vi "Add Data Sharing Framework with UDP Component to System Definition.vi"() -> ()   [LabVIEW 2017]
uses:
  DSF Core.lvlibp/Typedefs/DSF Engine Framework Configuration.ctl
  DSF Core.lvlibp/Typedefs/DSF Engine Plugin Configuration.ctl
  DSF Core.lvlibp/Typedefs/Core Plugin Configuration.ctl
  DSF Core.lvlibp/Typedefs/DSF Timing Info.ctl
  DSF Core.lvlibp/Typedefs/DSF Settings Info.ctl
  DSF Core.lvlibp/Typedefs/DSF Engine Plugin Thread Configuration.ctl
  DSF Core.lvlibp/Typedefs/Core Thread Configuration.ctl
  DSF Core.lvlibp/Typedefs/DSF Engine Transfer Group Configuration.ctl
  DSF Core.lvlibp/Typedefs/Core Group Configuration.ctl
  DSF Core.lvlibp/Typedefs/DSF Direction.ctl
  DSF Core.lvlibp/Typedefs/DSF Timeout Behavior.ctl
  DSF Core.lvlibp/Typedefs/DSF Engine Transfer Configuration.ctl
  DSF Core.lvlibp/Typedefs/Core Transfer Configuration.ctl
  DSF Core.lvlibp/Typedefs/DSF Engine Channel Configuration.ctl
  DSF Core.lvlibp/Typedefs/Core Channel Configuration.ctl
  DSF Core.lvlibp/Typedefs/DSF Data Type.ctl
  NationalInstruments.VeriStand.SystemDefinitionAPI
  DSF Core.lvlibp
  DSF Core.lvlibp/Classes/Configuration/Core/Channel/Channel Configuration.lvclass
  DSF Core.lvlibp/Classes/Configuration/Core/Transfer/Transfer Configuration.lvclass
  DSF Core.lvlibp/Classes/Configuration/Core/Group/Group Configuration.lvclass
  DSF Core.lvlibp/Classes/Configuration/Core/Thread/Thread Configuration.lvclass
  DSF Core.lvlibp/Classes/Configuration/Core/Plugin/Plugin Configuration.lvclass
  Scripting API/Data Sharing Framework Custom Device Scripting.lvlib
panel:
  in  "Launch Data Viewer":bool=TRUE
  in  "Data Server Frequency":dbl(ring)=10.0 items=["0.5 Hz"=0.5, "1.0 Hz"=1.0, "2.0 Hz"=2.0, "2.5 Hz"=2.5, "4.0 Hz"=4.0, "5.0 Hz"=5.0, "8.0 Hz"=8.0, "10.0 Hz"=10.0, "12.5 Hz"=12.5, "20.0 Hz"=20.0, "25.0 Hz"=25.0, "40.0 Hz"=40.0, "50.0 Hz"=50.0, "100.0 Hz"=100.0]
  in  "Enable Data Server":bool=TRUE
  in  "Channels":T1(array[cluster])
  in  "Output System Definition File":path=path "System Definition Files/DSF_UDP.nivssdf"
  in  "Input System Definition File":path=path "System Definition Files/DSF_empty.nivssdf"
  # "Overview: Demonstrates using the Data Sharing Framework scripting API to add a UDP plugin for data communication. \n\nInstructions:\n1. Per your application requirements, configure the data block to share.\n2. Browse to a path to save the system definition file as the output Output System Definition File.  This may be the same as the input file.\n3. Run the VI and verify its results."
  # "Configure Data Server for Validation"
  # "Data Sharing Framework Channels"
  # "System Definition Files"
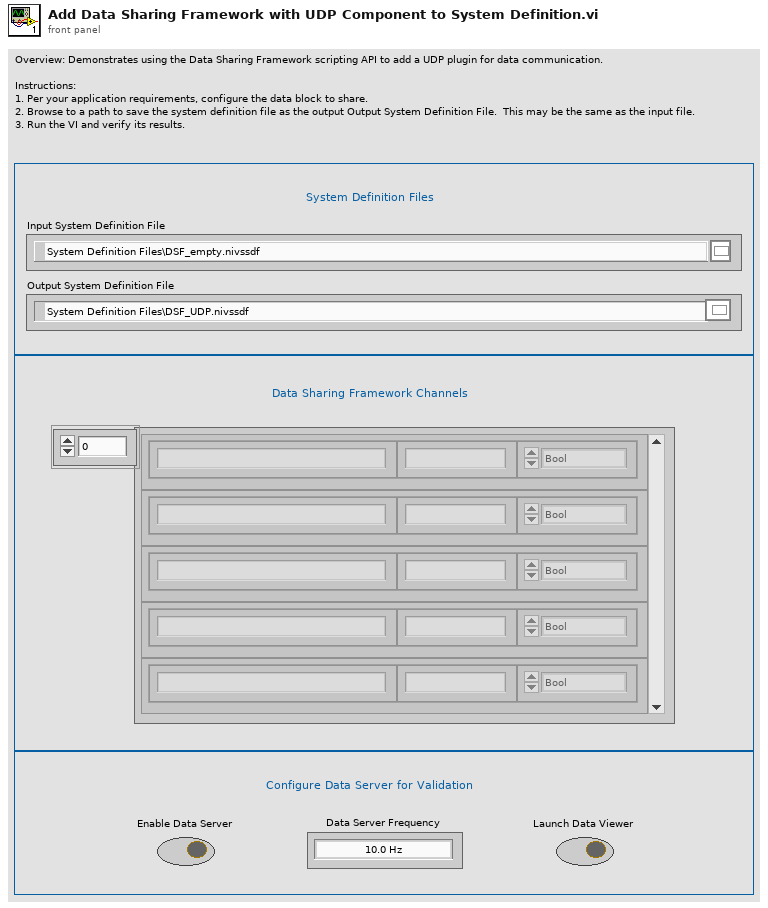
[diagram p1: front panel]
types:
  T1 = cluster{"Name":string, "Unit":string, "Buffer Datatype":enum16{"Bool", "SGL", "DBL", "I8", "I16", "I32", "I64", "U8", "U16", "U32", "U64"}}[]
  T2 = typedef "DSF Core.lvlibp/DSF Engine Channel Configuration.ctl" = cluster{"core":T3, "component settings":T5[]}
  T3 = typedef "DSF Core.lvlibp/Channel Configuration.lvclass/Core Channel Configuration.ctl" = cluster{"name":string, "units":string, "engine data type":T4, "string data type":T4, "string offset":u64}
  T4 = typedef "DSF Core.lvlibp/DSF Data Type.ctl" = enum8{"Bool", "SGL", "DBL", "I8", "I16", "I32", "I64", "U8", "U16", "U32", "U64"}
  T5 = typedef "DSF Core.lvlibp/DSF Settings Info.ctl" = cluster{"component":string, "values":cluster{"key":string, "value":string}[]}
  T6 = typedef "DSF Core.lvlibp/DSF Engine Plugin Thread Configuration.ctl" = cluster{"core":T7, "component settings":T5[], "transfer groups":T8[]}
  T7 = typedef "DSF Core.lvlibp/Thread Configuration.lvclass/Core Thread Configuration.ctl" = cluster{"processor":i32, "priority offset":i16}
  T8 = typedef "DSF Core.lvlibp/DSF Engine Transfer Group Configuration.ctl" = cluster{"core":T9, "component settings":T5[], "transfers":T13[]}
  T9 = typedef "DSF Core.lvlibp/Group Configuration.lvclass/Core Group Configuration.ctl" = cluster{"name":string, "direction":T10, "cycle timing":T11, "timeout behavior":T12, "enable conversion":bool}
  T10 = typedef "DSF Core.lvlibp/DSF Direction.ctl" = enum8{"Tx", "Rx"}
  T11 = typedef "DSF Core.lvlibp/DSF Timing Info.ctl" = cluster{"priority":u64, "decimation":u64, "offset":u64}
  T12 = typedef "DSF Core.lvlibp/DSF Timeout Behavior.ctl" = enum8{"Increment Late Count", "Throw Error"}
  T13 = typedef "DSF Core.lvlibp/DSF Engine Transfer Configuration.ctl" = cluster{"core":T14, "component settings":T5[], "channels":T2[]}
  T14 = typedef "DSF Core.lvlibp/Transfer Configuration.lvclass/Core Transfer Configuration.ctl" = cluster{"name":string}
  T15 = typedef "DSF Core.lvlibp/DSF Engine Plugin Configuration.ctl" = cluster{"core":T16, "component settings":T5[], "threads":T6[]}
  T16 = typedef "DSF Core.lvlibp/Plugin Configuration.lvclass/Core Plugin Configuration.ctl" = cluster{"name":string, "components":string[], "cycle timing":T11}
  T17 = typedef "DSF Core.lvlibp/DSF Engine Framework Configuration.ctl" = cluster{"plugins":T15[]}
  T18 = enum16{"Bool", "SGL", "DBL", "I8", "I16", "I32", "I64", "U8", "U16", "U32", "U64"}
  T19 = typedef "Custom Device API.lvlib/Custom Device Item Ref.ctl" = u64
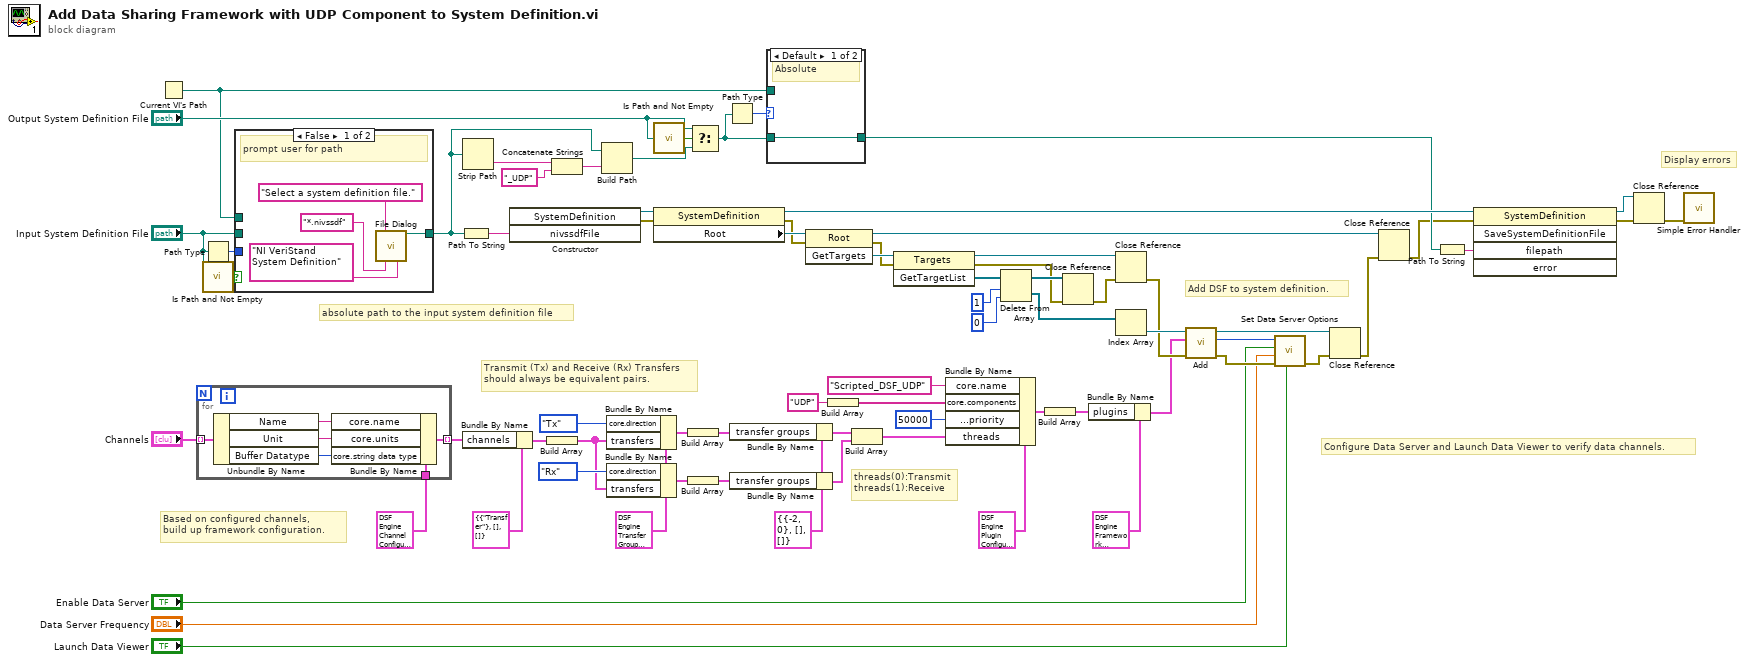
[diagram p0: block diagram]
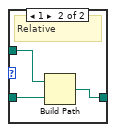
[diagram p2: hidden frame]
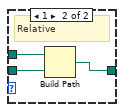
[diagram p4: hidden frame]
diagram:
  w21 = T6 {"core"={"processor"=-2, "priority offset"=0}, "component settings"=[], "transfer groups"=[]} ("element")
  w28 = T8 {"core"={"name"="Group", "direction"=enum."Tx", "cycle timing"={"priority"=100, "decimation"=1, "offset"=0}, "timeout behavior"=enum."Increment Late Count", "enable conversion"=FALSE}, "component settings"=[], "transfers"=[]} ("element")
  # "Transmit (Tx) and Receive (Rx) Transfers \nshould always be equivalent pairs."
  # "absolute path to the input system definition file"
  # "Display errors"
  # "Add DSF to system definition."
  # "threads(0):Transmit\nthreads(1):Receive"
  # "Based on configured channels, \nbuild up framework configuration."
  # "Configure Data Server and Launch Data Viewer to verify data channels."
  n1 = Current VI's Path() -> (path=w1:path)
  n2 = for {
    tunnel: "Channels" -> [w78] mode=indexing
    tunnel: [w74] -> w32 mode=indexing
    tunnel: T2 {"core"={"name"="Voltage", "units"="V", "engine data type"=enum."DBL", "string data type"=enum."DBL", "string offset"=0}, "component settings"=[]} ("channel configuration") -> [w73]
    n3 = Unbundle By Name(w78) -> ("Name"=w77:string, "Unit"=w76:string, "Buffer Datatype"=w75:T18)
    n4 = Bundle By Name(cluster=w73, "core.name"=w77, "core.units"=w76, "core.string data type"=w75) -> (w74:T2)
  }
  n5 = Path Type(1:"Input System Definition File") -> (0:w72:i16)
  n6 = call <vilib>:"Is Path and Not Empty.vi"("path"="Input System Definition File") -> ("Is Path and Not Empty?"=w70:bool)  [unwired: 4 in]
  n7 = case shown="False" w70 {
    tunnel: w72 -> [_ w86]
    tunnel: "Input System Definition File" -> [_ w85]
    tunnel: [w79 w84] -> w8
    tunnel: w1 -> [_ w83]
    frame False {
      # "prompt user for path"
      n8 = call "File Dialog"("prompt"="Select a system definition file.", "pattern (all files)"="*.nivssdf", "pattern label"="NI VeriStand System Definition") -> ("selected path"=w79:path)  [unwired: 9 in, 3 out]
    }
    frame True {
      # "input path converted to absolute"
      n9 = case shown="Default" w86 {
        tunnel: w83 -> [_ w90]
        tunnel: w85 -> [w87 w89]
        tunnel: [w87 w88] -> w84
        frame Default {
          # "Absolute"
        }
        frame 1 {
          # "Relative"
          n10 = Build Path(base path=w90, name or relative path=w89) -> (appended path=w88:path)
        }
      }
    }
  }
  n11 = Path To String(path=w8) -> (string=w55:string)
  n12 = Strip Path(path=w8) -> (name=w52:string)  [unwired: 1 out]
  n13 = Bundle By Name(cluster=T13 {"core"={"name"="Transfer"}, "component settings"=[], "channels"=[]} ("output cluster"), "channels"=w32) -> (w30:T13)
  n14 = constructor class="SystemDefinition"("nivssdfFile"=w55) -> (reference out=w57:refnum<k24>, error out=w56:errorcluster)  [unwired: 3 in, 2 out]
  n15 = Build Array(w30) -> (w29:T13[])
  n16 = Concatenate Strings(w52, "_UDP" ("string")) -> (w50:string)
  n17 = Build Path(base path=w8, name or relative path=w50) -> (appended path=w3:path)
  n18 = Bundle By Name(cluster=w28, "core.direction"=DSF_Direction."Tx", "transfers"=w29) -> (w27:T8)
  n19 = Bundle By Name(cluster=w28, "core.direction"=DSF_Direction."Rx", "transfers"=w29) -> (w26:T8)
  n20 = call <vilib>:"Is Path and Not Empty.vi"("path"="Output System Definition File") -> ("Is Path and Not Empty?"=w53:bool)  [unwired: 4 in]
  n21 = property class="SystemDefinition"(reference=w57, error in=w56) -> (reference out=w45:refnum<k24>, error out=w58:errorcluster, "Root"=w59:refnum<k24>)
  n22 = Build Array(w27) -> (w24:T8[])
  n23 = Build Array(w26) -> (w25:T8[])
  n24 = Select(t="Output System Definition File", s=w53, f=w3) -> (s? t:f=w49:path)
  n25 = Path Type(1:w49) -> (0:w54:i16)
  n26 = Bundle By Name(cluster=w21, "transfer groups"=w24) -> (w23:T6)
  n27 = Bundle By Name(cluster=w21, "transfer groups"=w25) -> (w22:T6)
  n28 = case shown="Default" w54 {
    tunnel: w1 -> [_ w94]
    tunnel: w49 -> [w91 w93]
    tunnel: [w91 w92] -> w41
    frame Default {
      # "Absolute"
    }
    frame 1 {
      # "Relative"
      n29 = Build Path(base path=w94, name or relative path=w93) -> (appended path=w92:path)
    }
  }
  n30 = invoke class="Root" method="GetTargets"(reference=w59, error in=w58) -> (reference out=w47:refnum<k24>, error out=w60:errorcluster, "GetTargets"=w61:refnum<k24>)  [unwired: 1 in]
  n31 = Build Array("UDP" ("class")) -> (w37:string[])
  n32 = Build Array(w23, w22) -> (w20:T6[])
  n33 = invoke class="Targets" method="GetTargetList"(reference=w61, error in=w60) -> (reference out=w68:refnum<k24>, error out=w65:errorcluster, "GetTargetList"=w62:refnum<k24>[])  [unwired: 1 in]
  n34 = Bundle By Name(cluster=T15 {"core"={"name"="", "components"=["UDP"], "cycle timing"={"priority"=10000, "decimation"=1, "offset"=0}}, "component settings"=[], "threads"=[{"core"={"processor"=-2, "priority offset"=0}, "component settings"=[], "transfer groups"=[{"core"={"name"="Group", "direction"=enum."Tx", "cycle timing"={"priority"=100, "decimation"=1, "offset"=0}, "timeout behavior"=enum."Increment Late Count", "enable conversion"=FALSE}, "component settings"=[], "transfers"=[{"core"={"name"="Transfer"}, "component settings"=[], "channels"=[{"core"={"name"="Voltage", "units"="V", "engine data type"=enum."DBL", "string data type"=enum."DBL", "string offset"=0}, "component settings"=[]}, {"core"={"name"="Current", "units"="A", "engine data type"=enum."DBL", "string data type"=enum."DBL", "string offset"=0}, "component settings"=[]}]}]}]}, {"core"={"processor"=-2, "priority offset"=0}, "component settings"=[], "transfer groups"=[{"core"={"name"="Group", "direction"=enum."Rx", "cycle timing"={"priority"=100, "decimation"=1, "offset"=0}, "timeout behavior"=enum."Increment Late Count", "enable conversion"=FALSE}, "component settings"=[], "transfers"=[{"core"={"name"="Transfer"}, "component settings"=[], "channels"=[{"core"={"name"="Voltage", "units"="V", "engine data type"=enum."DBL", "string data type"=enum."DBL", "string offset"=0}, "component settings"=[]}, {"core"={"name"="Current", "units"="A", "engine data type"=enum."DBL", "string data type"=enum."DBL", "string offset"=0}, "component settings"=[]}]}]}]}]} ("Plugin Configuration"), "core.name"="Scripted_DSF_UDP", "core.components"=w37, "core.cycle timing.priority"=u64 50000, "threads"=w20) -> (w19:T15)
  n35 = Delete From Array(array=w62, length=1, index=0) -> (deleted portion=w69:refnum<k24>[], array with subset deleted=w66:refnum<k24>[])
  n36 = Build Array(w19) -> (w17:T15[])
  n37 = Close Reference(reference=w66, error in (no error)=w65) -> (error out=w67:errorcluster)
  n38 = Bundle By Name(cluster=T17 {"plugins"=[{"core"={"name"="", "components"=["UDP"], "cycle timing"={"priority"=10000, "decimation"=1, "offset"=0}}, "component settings"=[], "threads"=[{"core"={"processor"=-2, "priority offset"=0}, "component settings"=[], "transfer groups"=[{"core"={"name"="Group", "direction"=enum."Tx", "cycle timing"={"priority"=100, "decimation"=1, "offset"=0}, "timeout behavior"=enum."Increment Late Count", "enable conversion"=FALSE}, "component settings"=[], "transfers"=[{"core"={"name"="Transfer"}, "component settings"=[], "channels"=[{"core"={"name"="Voltage", "units"="V", "engine data type"=enum."DBL", "string data type"=enum."DBL", "string offset"=0}, "component settings"=[]}, {"core"={"name"="Current", "units"="A", "engine data type"=enum."DBL", "string data type"=enum."DBL", "string offset"=0}, "component settings"=[]}]}]}]}, {"core"={"processor"=-2, "priority offset"=0}, "component settings"=[], "transfer groups"=[{"core"={"name"="Group", "direction"=enum."Rx", "cycle timing"={"priority"=100, "decimation"=1, "offset"=0}, "timeout behavior"=enum."Increment Late Count", "enable conversion"=FALSE}, "component settings"=[], "transfers"=[{"core"={"name"="Transfer"}, "component settings"=[], "channels"=[{"core"={"name"="Voltage", "units"="V", "engine data type"=enum."DBL", "string data type"=enum."DBL", "string offset"=0}, "component settings"=[]}, {"core"={"name"="Current", "units"="A", "engine data type"=enum."DBL", "string data type"=enum."DBL", "string offset"=0}, "component settings"=[]}]}]}]}]}]} ("framework configuration"), "plugins"=w17) -> (w7:T17)
  n39 = Close Reference(reference=w68, error in (no error)=w67) -> (error out=w10:errorcluster)
  n40 = Index Array(array=w69) -> (element=w13:refnum<k24>)  [unwired: 1 in]
  n41 = call "Add.vi"("error in"=w10, "framework configuration"=w7, "target in"=w13) -> ("error out"=w11:errorcluster, "data sharing framework custom device"=w14:T19, "target out"=w12:refnum<k24>)  [unwired: 6 in]
  n42 = call "Set Data Server Options.vi"("launch data viewer"="Launch Data Viewer", "error in"=w11, "data server frequency (Hz)"="Data Server Frequency", "enable data server"="Enable Data Server", "data sharing framework custom device in"=w14) -> ("error out"=w9:errorcluster)  [unwired: 4 in, 2 out]
  n43 = Close Reference(reference=w12, error in (no error)=w9) -> (error out=w48:errorcluster)
  n44 = Close Reference(reference=w47, error in (no error)=w48) -> (error out=w40:errorcluster)
  n45 = Path To String(path=w41) -> (string=w46:string)
  n46 = invoke class="SystemDefinition" method="SaveSystemDefinitionFile"(reference=w45, error in=w40, "filepath"=w46) -> (reference out=w43:refnum<k24>, error out=w44:errorcluster)  [unwired: 2 in, 3 out]
  n47 = Close Reference(reference=w43, error in (no error)=w44) -> (error out=w42:errorcluster)
  n48 = call <vilib>:"Simple Error Handler.vi"("error in (no error)"=w42) -> ()  [unwired: 1 in, 8 out]
